vi "Distributor - SET -  Actor_Name.vi"(8 "error in (no error)":errorcluster, 10 "Actor_Name":string, 11 "Parent_Class in":refnum<class "Message_Distributor_Class.lvclass">) -> (0 "error out":errorcluster, 3 "Parent_Class out":refnum<class "Message_Distributor_Class.lvclass">)   [LabVIEW 2023, in "Actor_Message_Distributor.lvlib" / "Message_Distributor_Class.lvclass"]
uses:
  Message_Distributor_Class.lvclass
  Message_Distributor_Class.lvclass/Message_Distributor_Class.ctl
  <vilib>/Utility/error.llb/Trim Whitespace One-Sided.vi
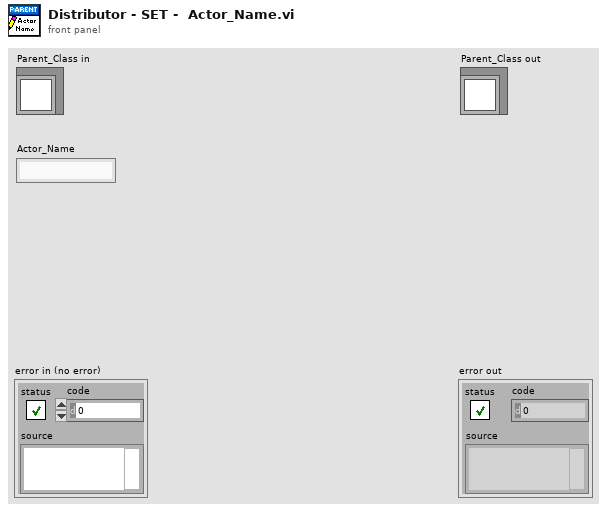
[diagram p1: front panel]
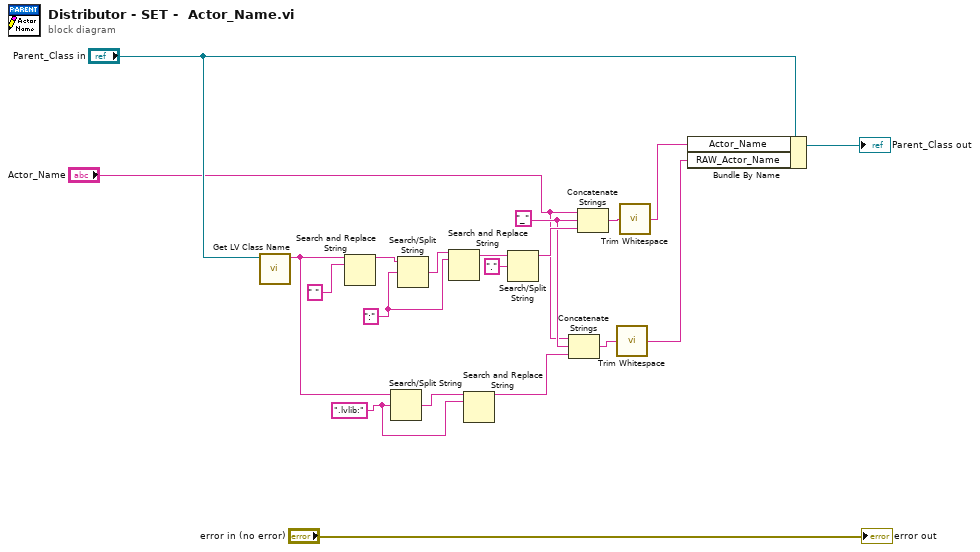
[diagram p0: block diagram]
diagram:
  w8 = ".lvlib:" ("search string/char (-)")
  w15 = ":" ("search string/char (-)")
  w5 = "_" ("string")
  n1 = call <vilib>:"Get LV Class Name.vi"("object"="Parent_Class in") -> ("class name"=w6:string)  [unwired: 9 in, 1 out]
  n2 = Search and Replace String(input string=w6, search string=" ") -> (result string=w17:string)  [unwired: 6 in, 3 out]
  n3 = Search/Split String(string=w6, search string/char (-)=w8) -> (match + rest of string=w7:string)  [unwired: 1 in, 2 out]
  n4 = Search/Split String(string=w17, search string/char (-)=w15) -> (match + rest of string=w16:string)  [unwired: 1 in, 2 out]
  n5 = Search and Replace String(input string=w16, search string=w15) -> (result string=w13:string)  [unwired: 6 in, 3 out]
  n6 = Search and Replace String(input string=w7, search string=w8) -> (result string=w3:string)  [unwired: 6 in, 3 out]
  n7 = Search/Split String(string=w13, search string/char (-)=".") -> (substring before match=w11:string)  [unwired: 1 in, 2 out]
  n8 = Concatenate Strings("Actor_Name", w5, w3) -> (w2:string)
  n9 = Concatenate Strings("Actor_Name", w5, w11) -> (w14:string)
  n10 = call <vilib>:"Trim Whitespace.vi"("string"=w2) -> ("trimmed string"=w1:string)  [unwired: 1 in]
  n11 = call <vilib>:"Trim Whitespace.vi"("string"=w14) -> ("trimmed string"=w9:string)  [unwired: 1 in]
  n12 = Bundle By Name(cluster="Parent_Class in", "Actor_Name"=w9, "RAW_Actor_Name"=w1) -> (→"Parent_Class out":refnum<class "Message_Distributor_Class.lvclass">)
  "error out" <- "error in (no error)"
